vi "Display.vi"() -> ()   [LabVIEW 2016, in "Aerotech VIs.lvlib"]
uses:
  Aerotech VIs.lvlib
panel:
  in  "Disconnect?":bool
  in  "refresh interval (msec)":i32
  in  "stop":bool
  in  "Axis":u16(ring) items=["X", "Y", "Z", "U", "A", "B", "C", "D", "x", "y", "z", "u", "a", "b", "c", "d", "XX", "YY", "ZZ", "UU", "AA", "BB", "CC", "DD", "xx", "yy", "zz", "uu", "aa", "bb", "cc", "dd"]
  out "Status":string
  in  "Tab Control":T1(tab)
  out "Position Command":dbl
  out "Position Feedback":dbl
  out "Prog Pos Command":dbl
  out "Prog Pos Feedback":dbl
  out "Velocity Command":dbl
  out "Velocity Feedback":dbl
  out "Current Command":sgl
  out "Current Feedback":sgl
  out "Pos Fbk Auxiliary":dbl
  out "error out":errorcluster
  out "Analog Input 0":dbl
  out "Analog Input 1":dbl
  out "Digital Input":bool[](array[boolean])
  out "Digital Output":bool[](array[boolean])
  out "Axis Fault (bits)":T2
  out "Axis Status (bits)":T3
  out "Drive Status (bits)":T4
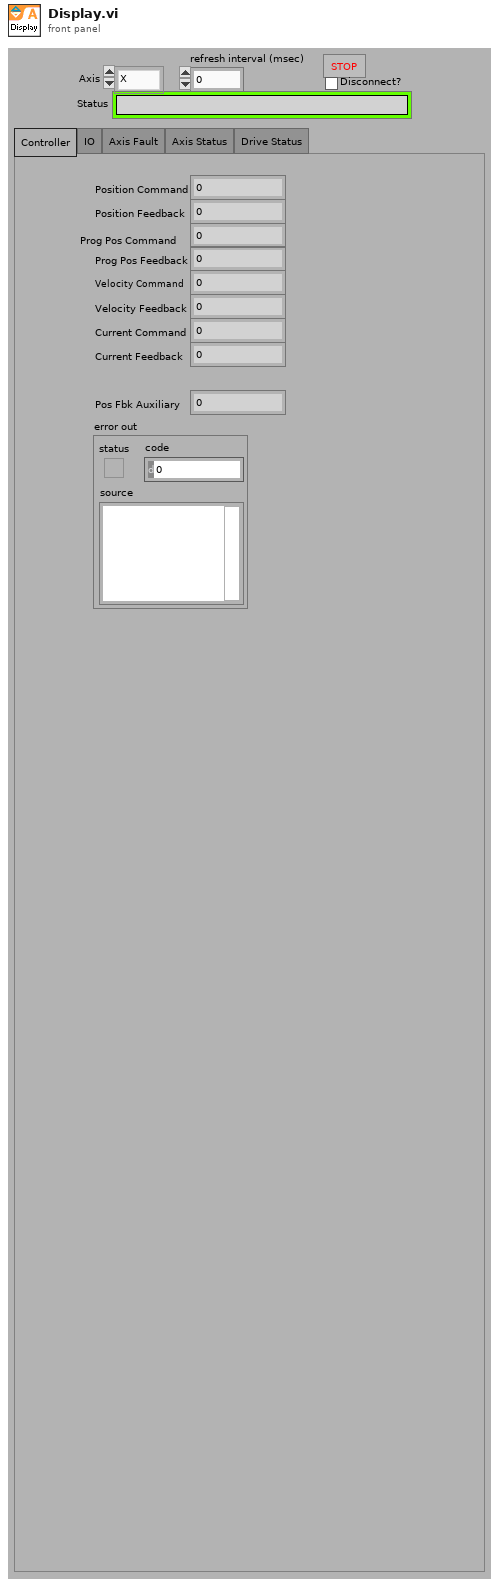
[diagram p1: front panel]
types:
  T1 = enum32{"Controller", "IO", "Axis Fault", "Axis Status", "Drive Status"}
  T2 = cluster{"AmplifierFault":bool, "AmplifierTemperatureFault":bool, "CcwEndOfTravelLimitFault":bool, "CcwSoftwareLimitFault":bool, "CommunicationLostFault":bool, "CwEndOfTravelLimitFault":bool, "CwSoftwareLimitFault":bool, "EmergencyStopFault":bool, "EncoderFault":bool, "ExternalFault":bool, "FeedbackScalingFault":bool, "GantryMisalignFault":bool, "HallSensorFault":bool, "InPositionTimeoutFault":bool, "MarkerSearchFault":bool, "MaxVelocityCommandFault":bool, "MotorTemperatureFault":bool, "None":bool, "OverCurrentFault":bool, "PositionErrorFault":bool, "PositionFeedbackFault":bool, "PowerSupplyFault":bool, "ProbeInputFault":bool, "SafeZoneFault":bool, "VelocityErrorFault":bool, "VelocityFeedbackFault":bool, "VoltageClampFault":bool}
  T3 = cluster{"BacklashActive":bool, "CalibrationEnabled1D":bool, "CalibrationEnabled2D":bool, "CommandValid":bool, "DriveAbortPending":bool, "DrivePending":bool, "Enabling":bool, "GainMappingEnabled":bool, "GantryAligned":bool, "GantryRealigning":bool, "Homed":bool, "Homing":bool, "IFOVEnabled":bool, "JogGenerating":bool, "Jogging":bool, "JoystickControl":bool, "MasterSlaveControl":bool, "MotionBlocked":bool, "MotionClamped":bool, "MoveDone":bool, "None":bool, "NotVirtual":bool, "Profiling":bool, "Stability0":bool, "Stability1":bool, "TrajectoryFiltering":bool, "WaitDone":bool}
  T4 = cluster{"AccelerationPhase":bool, "AutofocusActive":bool, "BrakeOutput":bool, "CcwEndOfTravelLimitInput":bool, "CosineEncoderError":bool, "CurrentClamp":bool, "CwEndOfTravelLimitInput":bool, "DecelerationPhase":bool, "DualLoopActive":bool, "EmergencyStopInput":bool, "Enabled":bool, "EncoderClipping":bool, "GalvoCalibrationEnabled":bool, "GalvoPowerCorrection":bool, "HallAInput":bool, "HallBInput":bool, "HallCInput":bool, "HighResolutionMode":bool, "HomeLimitInput":bool, "InPosition":bool, "InPosition2":bool, "MarkerInput":bool, "MarkerLatch":bool, "MoveActive":bool, "NoMotorSupply":bool, "None":bool, "PowerLimiting":bool, "ProgrammingFlash":bool, "ProgrammingMXH":bool, "PSOHaltLatch":bool, "ServoControl":bool, "SineEncoderError":bool}
  T5 = cluster{"new reference":refnum<k24>, "Event Callback":refnum<k27>, "ControllerDiagPacket":refnum<user-event>, "Event Registration Refnum":refnum<event-registration>}
  T6 = typedef "AxisDiagPacket.ctl" = cluster{"Axis Name":string, "Analog Input 0":dbl, "Analog Input 1":dbl, "Axis Fault (num)":i32, "Axis Fault (str)":string, "Axis Fault (bits)":cluster{"AmplifierFault":bool, "AmplifierTemperatureFault":bool, "CcwEndOfTravelLimitFault":bool, "CcwSoftwareLimitFault":bool, "CommunicationLostFault":bool, "CwEndOfTravelLimitFault":bool, "CwSoftwareLimitFault":bool, "EmergencyStopFault":bool, "EncoderFault":bool, "ExternalFault":bool, "FeedbackScalingFault":bool, "GantryMisalignFault ":bool, "HallSensorFault":bool, "InPositionTimeoutFault":bool, "MarkerSearchFault":bool, "MaxVelocityCommandFault":bool, "MotorTemperatureFault":bool, "None":bool, "OverCurrentFault":bool, "PositionErrorFault":bool, "PositionFeedbackFault":bool, "ProbeInputFault":bool, "SafeZoneFault":bool, "VelocityErrorFault":bool, "VelocityFeedbackFault":bool, "VoltageClampFault":bool, "PowerSupplyFault":bool}, "Axis Status (num)":i32, "Axis Status (str)":string, "Axis Status (bits)":cluster{"BacklashActive":bool, "CalibrationEnabled1D":bool, "CalibrationEnabled2D":bool, "CommandValid":bool, "DriveAbortPending":bool, "DrivePending":bool, "Enabling":bool, "GainMappingEnabled":bool, "GantryAligned":bool, "GantryRealigning":bool, "Homed":bool, "Homing":bool, "IFOVEnabled":bool, "Jogging":bool, "JogGenerating":bool, "JoystickControl":bool, "MasterSlaveControl":bool, "MotionBlocked":bool, "MotionClamped":bool, "MoveDone":bool, "None":bool, "NotVirtual":bool, "Profiling":bool, "Stability0":bool, "Stability1":bool, "TrajectoryFiltering":bool, "WaitDone":bool}, "Current Command":sgl, "Current Error":sgl, "Current Feedback":sgl, "Digital Inputs":i32, "Digital Outputs":i32, "Drive Status":i32, "Drive Status (str)":string, "Drive Status (bits)":cluster{"AccelerationPhase":bool, "AutofocusActive":bool, "BrakeOutput":bool, "CcwEndOfTravelLimitInput":bool, "CosineEncoderError":bool, "CurrentClamp":bool, "CwEndOfTravelLimitInput":bool, "DecelerationPhase":bool, "DualLoopActive":bool, "EmergencyStopInput":bool, "Enabled":bool, "EncoderClipping":bool, "GalvoCalibrationEnabled":bool, "GalvoPowerCorrection":bool, "HallAInput":bool, "HallBInput":bool, "HallCInput":bool, "HighResolutionMode":bool, "HomeLimitInput":bool, "InPosition":bool, "InPosition2":bool, "MarkerInput":bool, "MarkerLatch":bool, "MoveActive":bool, "NoMotorSupply":bool, "None":bool, "PowerLimiting":bool, "ProgrammingFlash":bool, "ProgrammingMXH":bool, "PSOHaltLatch":bool, "ServoControl":bool, "SineEncoderError":bool}, "Position Feedback Auxiliary":dbl, "Position Command":dbl, "Position Error":dbl, "Position Feedback":dbl, "Program Position Command":dbl, "Program Position Error":dbl, "Program Position Feedback":dbl, "Velocity Command":dbl, "Velocity Error":dbl, "Velocity Feedback":dbl}
  T7 = cluster{"AmplifierFault":bool, "AmplifierTemperatureFault":bool, "CcwEndOfTravelLimitFault":bool, "CcwSoftwareLimitFault":bool, "CommunicationLostFault":bool, "CwEndOfTravelLimitFault":bool, "CwSoftwareLimitFault":bool, "EmergencyStopFault":bool, "EncoderFault":bool, "ExternalFault":bool, "FeedbackScalingFault":bool, "GantryMisalignFault ":bool, "HallSensorFault":bool, "InPositionTimeoutFault":bool, "MarkerSearchFault":bool, "MaxVelocityCommandFault":bool, "MotorTemperatureFault":bool, "None":bool, "OverCurrentFault":bool, "PositionErrorFault":bool, "PositionFeedbackFault":bool, "ProbeInputFault":bool, "SafeZoneFault":bool, "VelocityErrorFault":bool, "VelocityFeedbackFault":bool, "VoltageClampFault":bool, "PowerSupplyFault":bool}
  T8 = cluster{"BacklashActive":bool, "CalibrationEnabled1D":bool, "CalibrationEnabled2D":bool, "CommandValid":bool, "DriveAbortPending":bool, "DrivePending":bool, "Enabling":bool, "GainMappingEnabled":bool, "GantryAligned":bool, "GantryRealigning":bool, "Homed":bool, "Homing":bool, "IFOVEnabled":bool, "Jogging":bool, "JogGenerating":bool, "JoystickControl":bool, "MasterSlaveControl":bool, "MotionBlocked":bool, "MotionClamped":bool, "MoveDone":bool, "None":bool, "NotVirtual":bool, "Profiling":bool, "Stability0":bool, "Stability1":bool, "TrajectoryFiltering":bool, "WaitDone":bool}
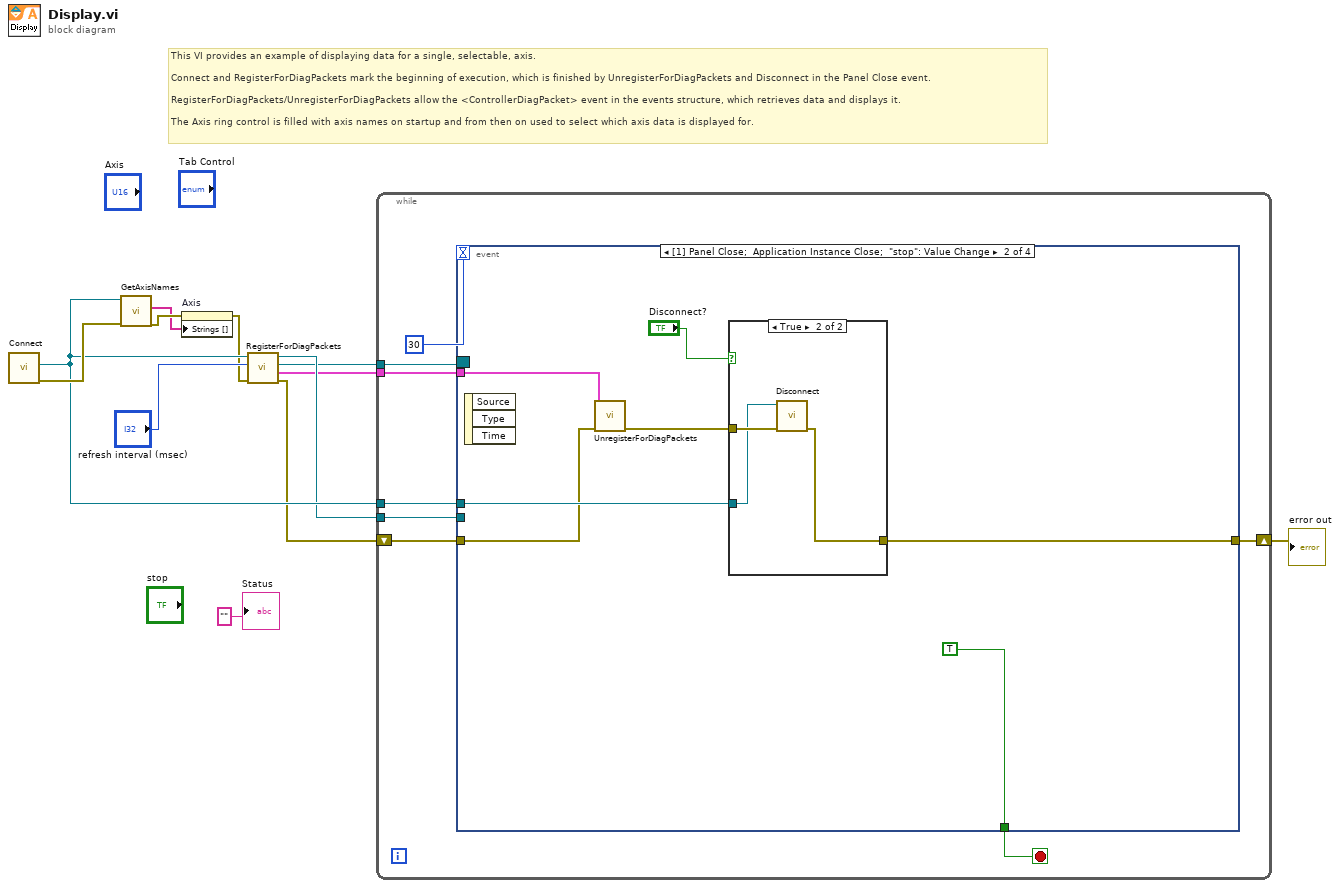
[diagram p0: block diagram]
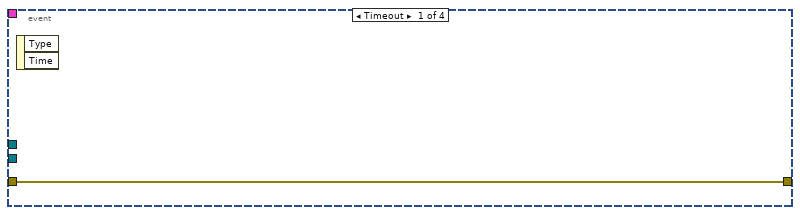
[diagram p2: hidden frame]
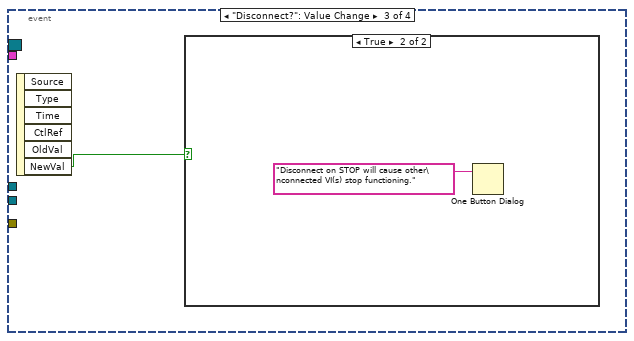
[diagram p4: hidden frame]
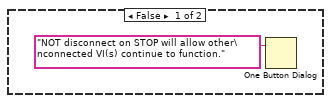
[diagram p5: hidden frame]
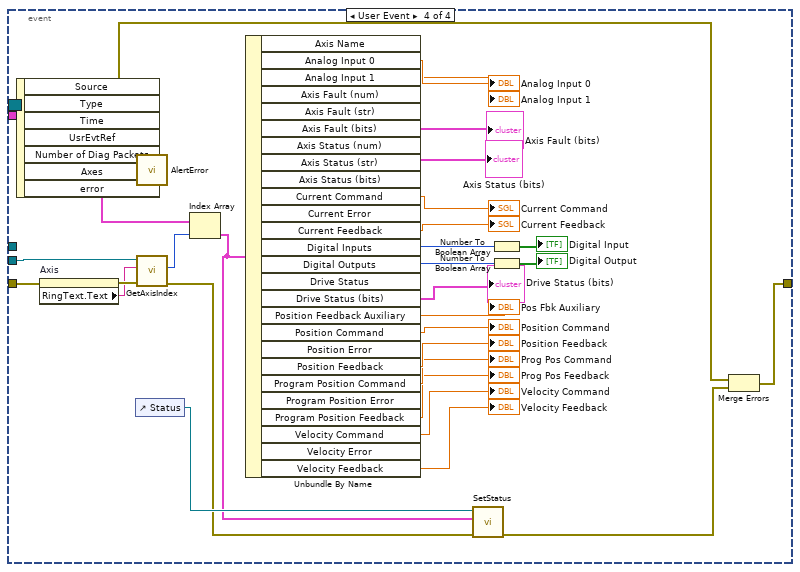
[diagram p6: hidden frame]
diagram:
  # "This VI provides an example of displaying data for a single, selectable, axis. \n\nConnect and RegisterForDiagPackets mark the beginning of execution, which is finished by UnregisterForDiagPackets and Disconnect in the Panel Close event.\n\nRegisterForDiagPackets/UnregisterForDiagPackets allow the <ControllerDiagPacket> event in the events structure, which retrieves data and displays it.\n\nThe Axis ring control is filled with axis names on startup and from then on used to select which axis data is displayed for."
  n1 = call "Connect.vi"() -> ("error out"=w10:errorcluster, "controller"=w7:refnum<k24>)  [unwired: 10 in]
  n2 = call "GetAxisNames.vi"("error in (no error)"=w10, "controller in"=w7) -> ("error out"=w11:errorcluster, "axis names"=w9:string[])  [unwired: 7 in, 1 out]
  n3 = property on="Axis" class="Ring (strict)"(error in=w11, "Strings []"=w9) -> (error out=w5:errorcluster)  [unwired: 1 in, 1 out]
  n4 = call "RegisterForDiagPackets.vi"("error in (no error)"=w5, "refresh interval (default)"="refresh interval (msec)", "Controller in"=w7) -> ("error out"=w2:errorcluster, "Event Metadata"=w1:T5, "Event Registration Refnum"=w3:refnum<event-registration>, "Controller out"=w4:refnum<k24>)  [unwired: 4 in]
  n5 = while {
    tunnel: w3 -> [w20]
    tunnel: w4 -> [w19]
    shift-right: [w15] -> w8
    shift-left: w2 -> [w18]
    tunnel: w7 -> [w14]
    tunnel: w1 -> [w13]
    stop <- w17 stop-if-true
    n6 = event shown="[1] Panel Close;  Application Instance Close;  \"stop\": Value Change" {
      selector: w20 -> [_ _ _ _]
      dyn-events: _ -> [_ _ _ _]
      timeout: 30 -> [_ _ _ _]
      tunnel: w19 -> [_ _ _ w59]
      tunnel: w18 -> [w21 w24 _ w58]
      tunnel: [_ TRUE _ _] -> w17
      tunnel: [w21 w27 _ w63] -> w15
      tunnel: w14 -> [_ w26 _ _]
      tunnel: w13 -> [_ w22 _ _]
      event Timeout {
        n7 = event-data() -> ()  [unwired: 1 in, 2 out]
      }
      event Panel Close; Application Instance Close; "stop": Value Change {
        n8 = event-data() -> ()  [unwired: 1 in, 3 out]
        n9 = call "UnregisterForDiagPackets.vi"("Event Metadata"=w22, "error in (no error)"=w24) -> ("error out"=w23:errorcluster)  [unwired: 8 in]
        n10 = case shown="True" "Disconnect?" {
          tunnel: w23 -> [w29 w32]
          tunnel: [w29 w31] -> w27
          tunnel: w26 -> [_ w30]
          frame False {
          }
          frame True {
            n11 = call "Disconnect.vi"("error in (no error)"=w32, "controller"=w30) -> ("error out"=w31:errorcluster)  [unwired: 9 in]
          }
        }
      }
      event "Disconnect?": Value Change {
        n12 = event-data() -> ("NewVal"=w33:bool)  [unwired: 1 in, 5 out]
        n13 = case shown="True" w33 {
          frame False {
            n14 = One Button Dialog(message="NOT disconnect on STOP will allow other\nconnected VI(s) continue to function.") -> ()  [unwired: 1 in, 1 out]
          }
          frame True {
            n15 = One Button Dialog(message="Disconnect on STOP will cause other\nconnected VI(s) stop functioning.") -> ()  [unwired: 1 in, 1 out]
          }
        }
      }
      event User Event {
        n16 = event-data() -> ("Axes"=w37:T6[], "error"=w62:errorcluster)  [unwired: 1 in, 5 out]
        n17 = property on="Axis" class="Ring (strict)"(error in=w58) -> (error out=w57:errorcluster, "RingText.Text"=w56:string)  [unwired: 1 in, 1 out]
        n18 = control-ref of="Status"() -> (w65:refnum<vi>)
        n19 = call "AlertError.vi"("error in (no error)"=w62) -> ()  [unwired: 10 in, 1 out]
        n20 = call "GetAxisIndex.vi"("error in (no error)"=w57, "axis name"=w56, "controller in"=w59) -> ("error out"=w55:errorcluster, "axis index"=w39:i32)  [unwired: 6 in, 1 out]
        n21 = Index Array(array=w37, index=w39) -> (element=w36:T6)
        n22 = Unbundle By Name(w36) -> ("Analog Input 0"=→"Analog Input 0":dbl, "Analog Input 1"=→"Analog Input 1":dbl, "Axis Fault (bits)"=→"Axis Fault (bits)":T7, "Axis Status (bits)"=→"Axis Status (bits)":T8, "Current Command"=→"Current Command":sgl, "Current Feedback"=→"Current Feedback":sgl, "Digital Inputs"=w52:i32, "Digital Outputs"=w51:i32, "Drive Status (bits)"=→"Drive Status (bits)":T4, "Position Feedback Auxiliary"=→"Pos Fbk Auxiliary":dbl, "Position Command"=→"Position Command":dbl, "Position Feedback"=→"Position Feedback":dbl, "Program Position Command"=→"Prog Pos Command":dbl, "Program Position Feedback"=→"Prog Pos Feedback":dbl, "Velocity Command"=→"Velocity Command":dbl, "Velocity Feedback"=→"Velocity Feedback":dbl)  [unwired: 10 out]
        n23 = call "SetStatus.vi"("error in (no error)"=w55, "AxisDiagPacket"=w36, "Status string"=w65) -> ("error out"=w64:errorcluster)  [unwired: 8 in]
        n24 = Number To Boolean Array(number=w52) -> (Boolean array=→"Digital Input":bool[])
        n25 = Number To Boolean Array(number=w51) -> (Boolean array=→"Digital Output":bool[])
        n26 = Merge Errors(w62, w64) -> (w63:errorcluster)
      }
    }
  }
  "error out" <- w8
  "Status" <- "" ("Status")
